vi "BBO2.vi"(6 "시작시간 값":u32, 8 "ROI 2":T1={"Global Rectangle"=[482, 445, 741, 571], "Contours"=[{"Contour Type"=0, "ROI Type"=3, "Points"=[482, 445, 741, 571]}]}, 9 "카메라 X":dbl=22.0, 10 "핀간격":dbl=40.0, 11 "클러스터":T2={{"정지할 차이값"=0.08, "흰색과 밖 차이값"=0.15, "흰/검 반 값 "=0.3}, {"4: 오른각도"=122.0, "4: 뒷쪽각도"=0.0, "5: 오른각도"=120.0, "5: 앞쪽각도"=245.0, "6: 왼쪽각도"=245.0, "6: 앞쪽각도"=120.0}, {"2: 공각도"=233.0, "2: 굴릴각도"=60.0}}) -> (3 "ROI":T1={"Global Rectangle"=[536, 448, 795, 574], "Contours"=[{"Contour Type"=0, "ROI Type"=3, "Points"=[536, 448, 795, 574]}]})   [LabVIEW 2014]
doc: "The myRIO Project template acquires acceleration data from the onboard accelerometer and displays the changes of acceleration values in a waveform chart."
uses:
  <vilib>/userdefined/High Color/IMAQdx.ctl
  <vilib>/vision/driver/NI_Vision_Acquisition_Software.lvlib
  <vilib>/vision/NI_Vision_Development_Module.lvlib
panel:
  out "시간체크":u32=10797
  in  "Range":cluster{"Lower value":sgl, "Upper value":sgl}={"Lower value"=128.0, "Upper value"=255.0} {"Upper value" format="%.2f"; "Lower value" format="%.2f"}
  in  "조정":dbl=100.0
  in  "수평(뒤로) 초":u32=150
  out "Number of Particles":i32=4
  in  "Local":T3={"Object Type"=0, "Method"=1, "Niblack Deviation Factor"=1.0, "Window"={"Width"=20, "Height"=20}} {"Niblack Deviation Factor" min=0.0 max=1.0 format="%.2f"; "Method" items=["Niblack", "Background Correction"]; "Object Type" items=["Bright Objects", "Dark Objects"]}
  out "숫자형 컨트롤":i32=11
  out "볼링핀을찾았는가":bool=TRUE
  in  "공 굴릴 범위":dbl=5.0
  in  "작게 움직이는 범위":dbl=500.0
  in  "좌우모터":i16=25
  out "Image 2":T4(plugin-control)
  out "Image":T4(plugin-control)
  # "Control Motor"
  # "Read Encoder"
  # "중간 22"
  # "25"
  # "1,3핀 12"
  # "1일때 + 0일때 -"
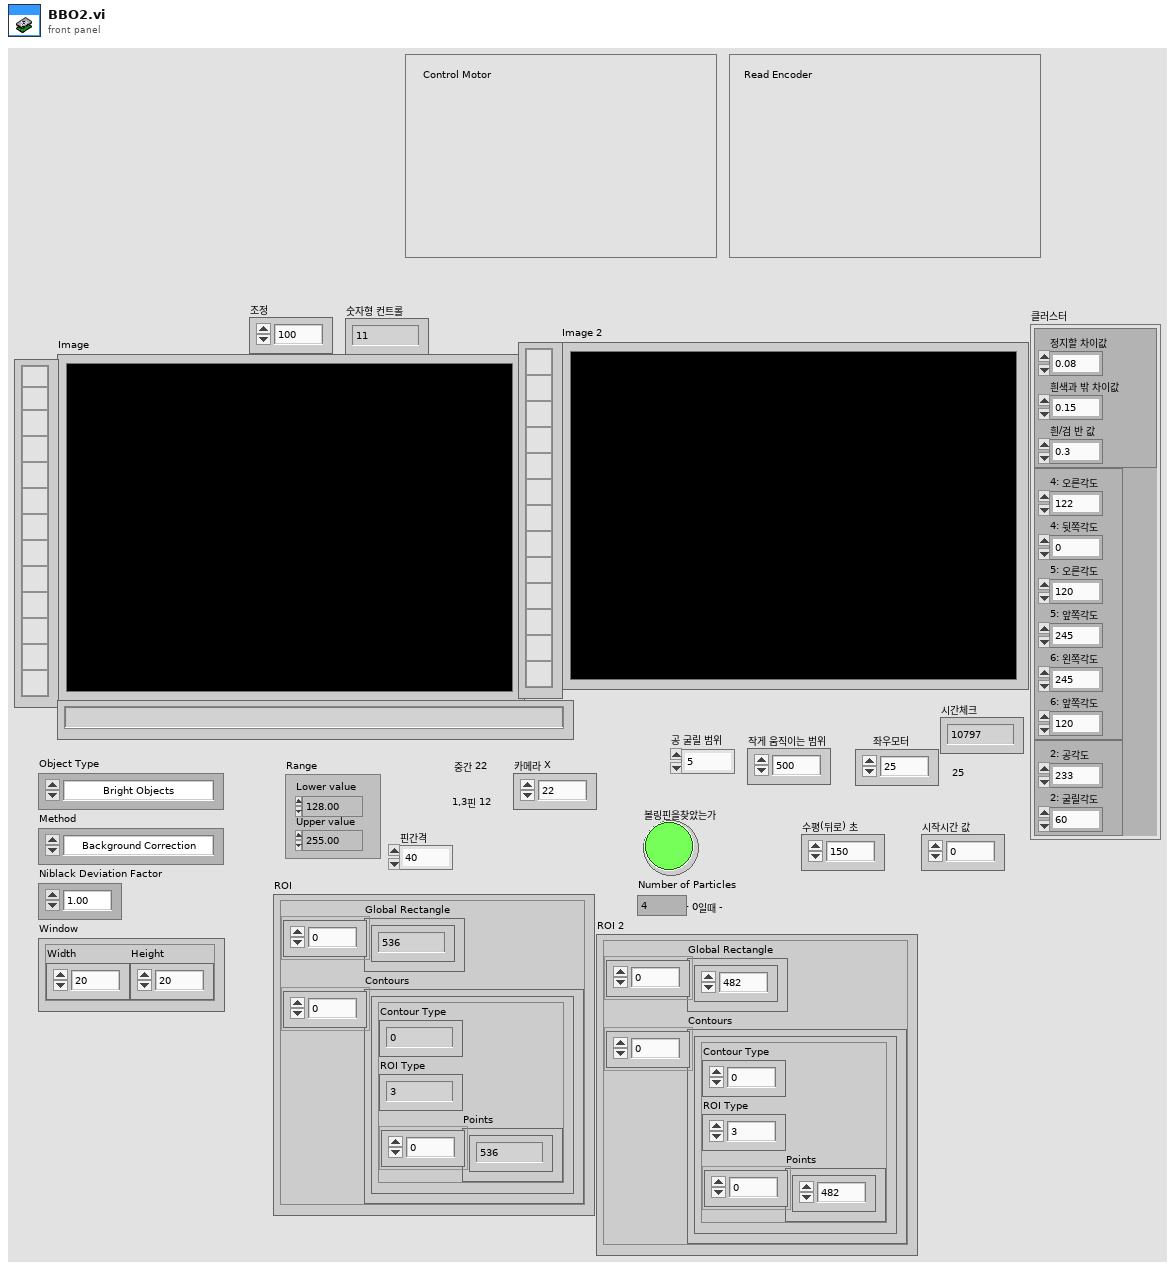
[diagram p1: front panel]
types:
  T1 = cluster{"Global Rectangle":i32[], "Contours":cluster{"Contour Type":u32, "ROI Type":u32, "Points":i32[]}[]}
  T2 = cluster{cluster{"정지할 차이값":dbl, "흰색과 밖 차이값":dbl, "흰/검 반 값 ":dbl}, cluster{"4: 오른각도":dbl, "4: 뒷쪽각도":dbl, "5: 오른각도":dbl, "5: 앞쪽각도":dbl, "6: 왼쪽각도":dbl, "6: 앞쪽각도":dbl}, cluster{"2: 공각도":dbl, "2: 굴릴각도":dbl}}
  T3 = cluster{"Object Type":u32, "Method":u32, "Niblack Deviation Factor":dbl, "Window":cluster{"Width":i32, "Height":i32}}
  T4 = typedef "IMAQ Image.ctl" = refnum<image>
  T5 = typedef "IMAQdx.ctl" = refnum<k21>
  T6 = typedef "IMAQ Rectangle" = cluster{"Left":i32, "Top":i32, "Right":i32, "Bottom":i32, "Rotation":dbl}
  T7 = cluster{"Niblack Deviation Factor":dbl, "Niblack Deviation Factor":dbl}
  T8 = typedef "Image Type" = u32
  T9 = cluster{"Area":dbl, "Number of Holes":dbl, "Bounding Rect":cluster{"Left":dbl, "Top":dbl, "Right":dbl, "Bottom":dbl}, "Center of Mass":cluster{"X":dbl, "Y":dbl}, "Orientation":dbl, "Dimensions":cluster{"Width":dbl, "Height":dbl}}[]
  T10 = cluster{"Left":dbl, "Top":dbl, "Right":dbl, "Bottom":dbl}
  T11 = typedef "ROI Descriptor" = cluster{"Global Rectangle":i32[], "Contours":cluster{"ID":enum32{"External", "Internal"}, "Type":u32, "Coordinates":i32[]}[]}
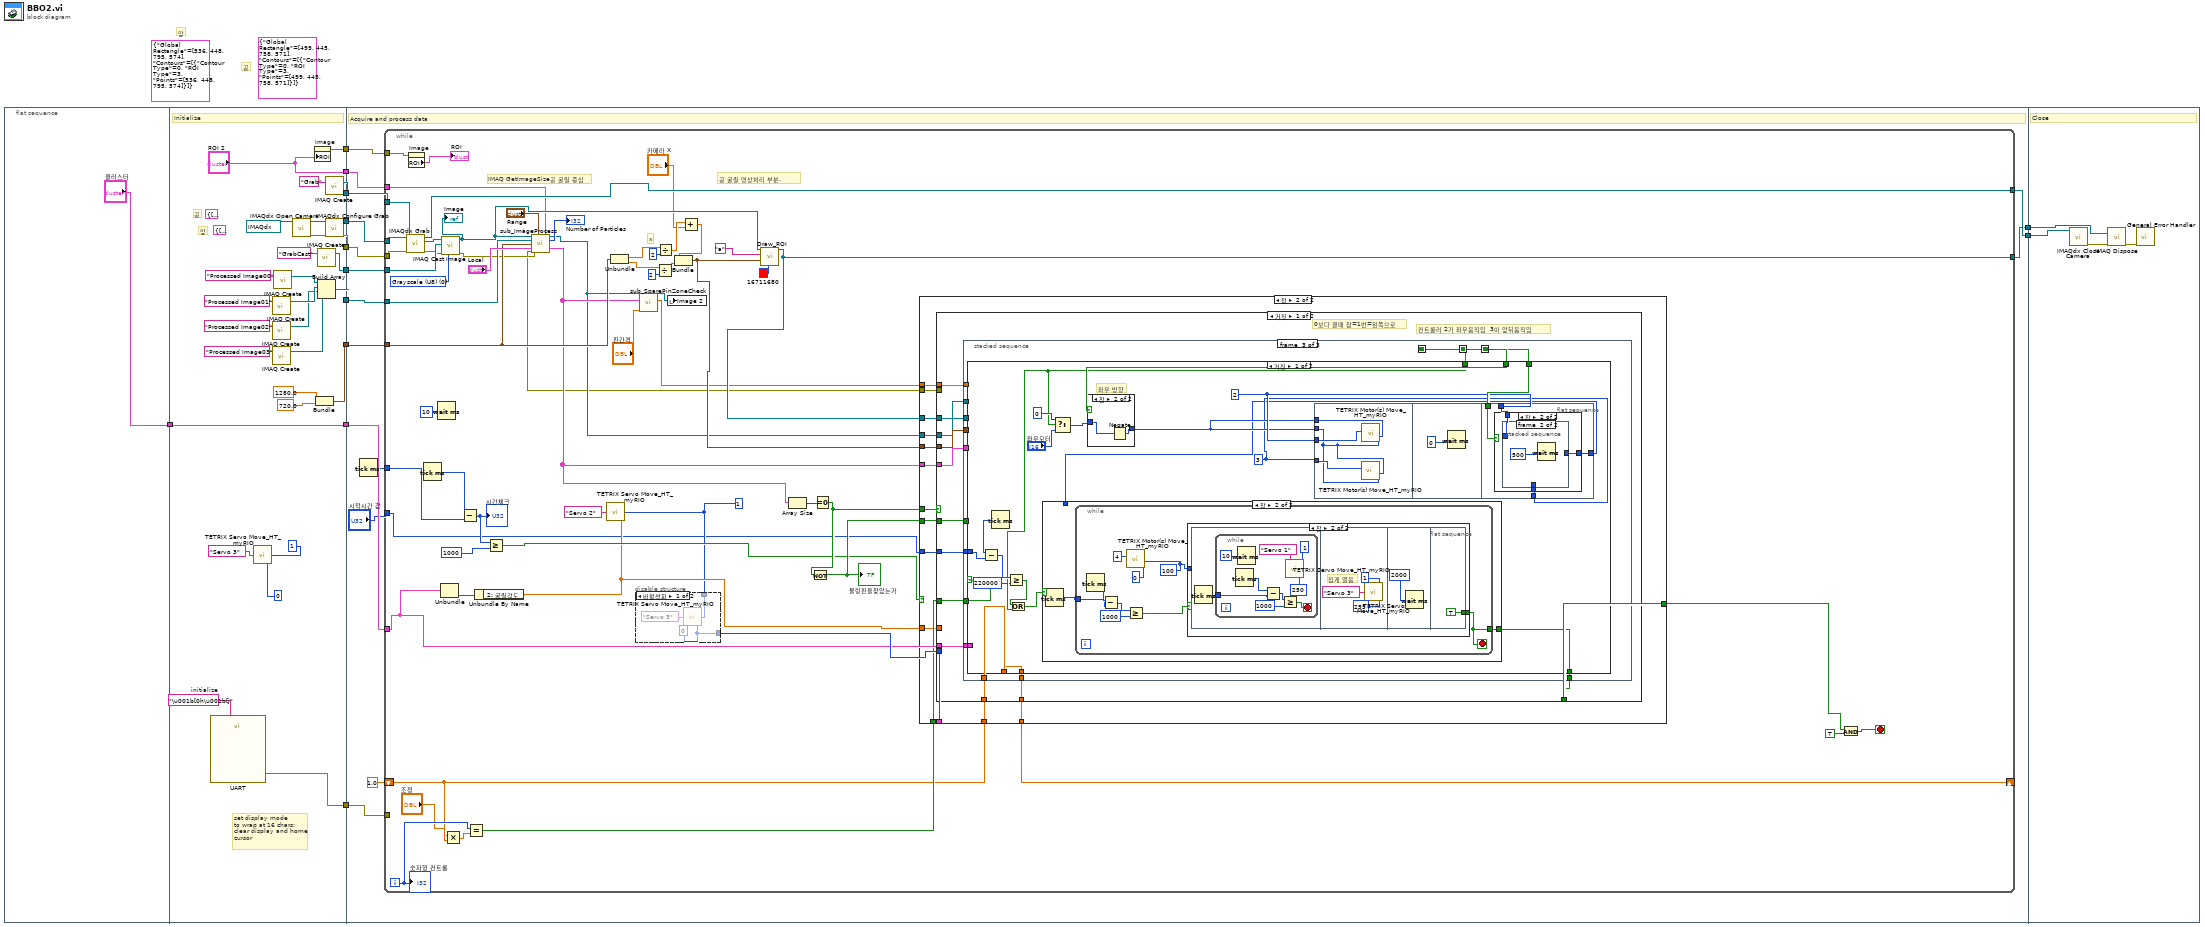
[diagram p0: block diagram]
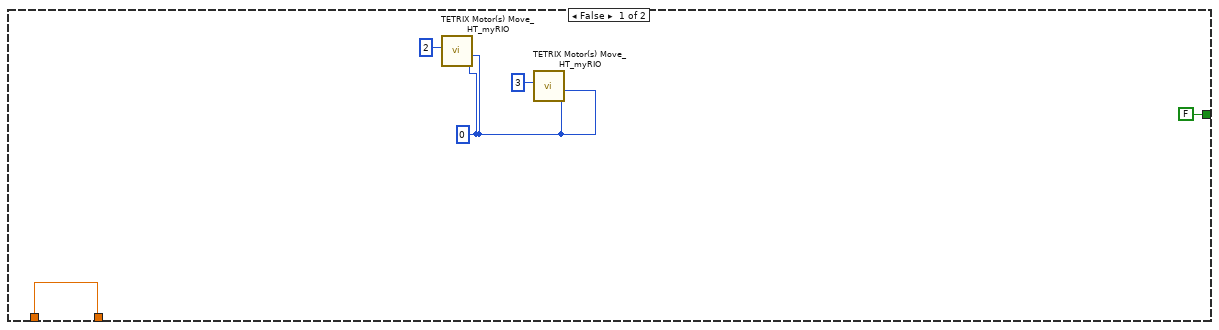
[diagram p3: hidden frame]
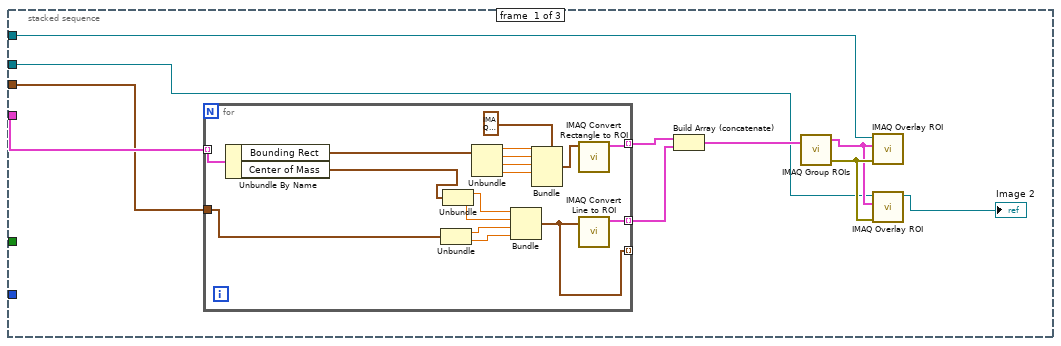
[diagram p4: hidden frame]
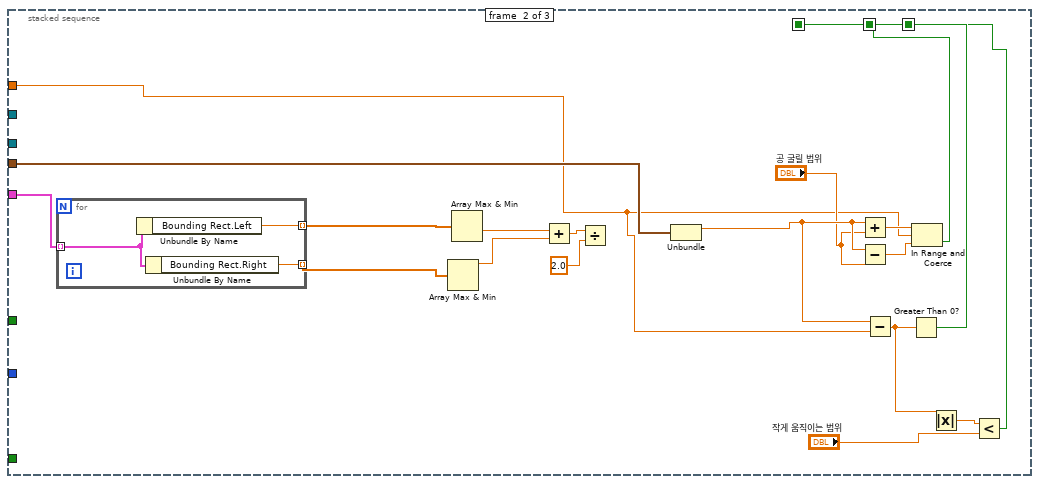
[diagram p5: hidden frame]
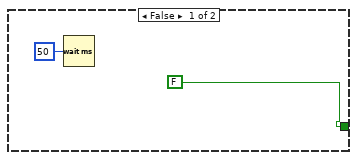
[diagram p6: hidden frame]
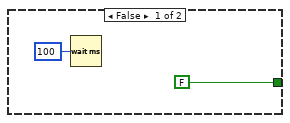
[diagram p7: hidden frame]
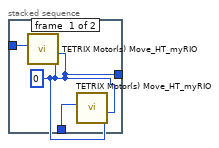
[diagram p9: hidden frame]
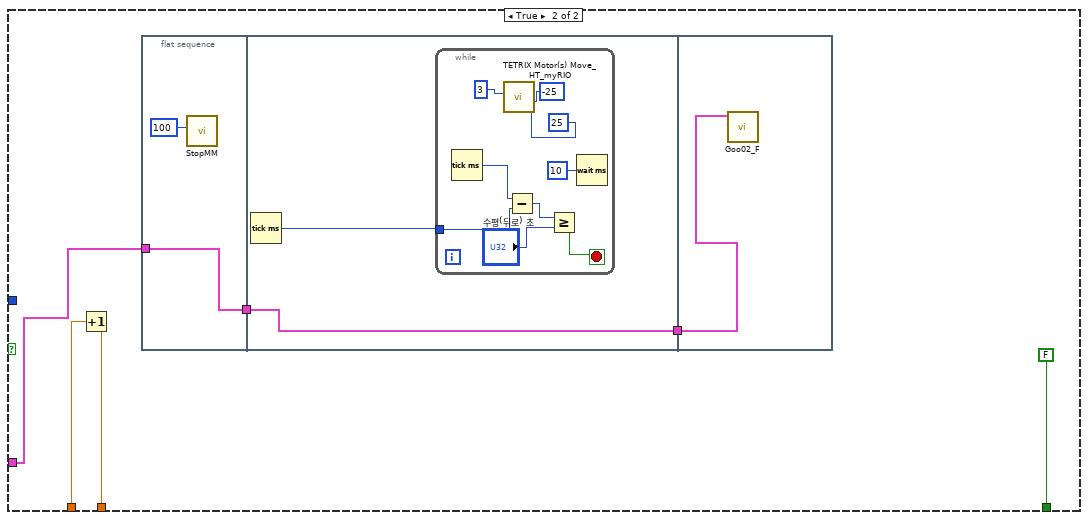
[diagram p11: hidden frame]
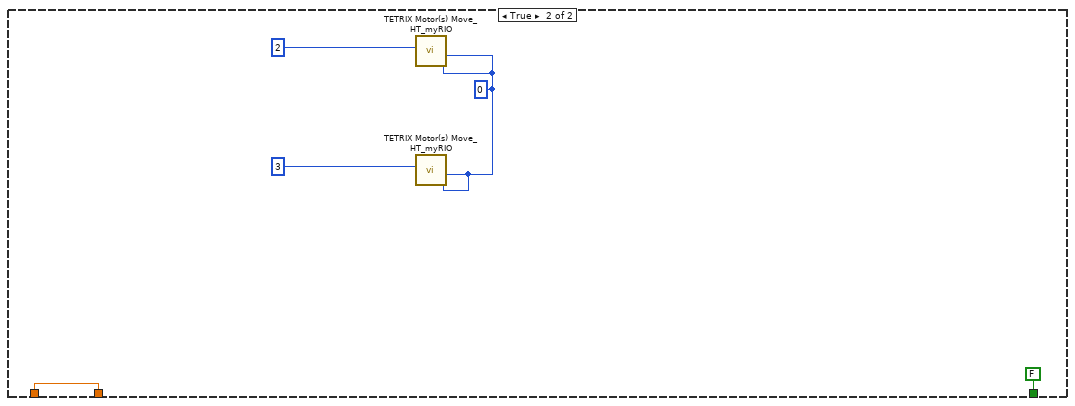
[diagram p12: hidden frame]
diagram:
  (unwired) T1 {"Global Rectangle"=[499, 445, 758, 571], "Contours"=[{"Contour Type"=0, "ROI Type"=3, "Points"=[499, 445, 758, 571]}]} ("ROI")
  (unwired) T1 {"Global Rectangle"=[536, 448, 795, 574], "Contours"=[{"Contour Type"=0, "ROI Type"=3, "Points"=[536, 448, 795, 574]}]} ("ROI")
  # "공"
  # "앞"
  n1 = flat-sequence {
    tunnel: ["클러스터"] -> w3
    tunnel: [w40] -> w13
    tunnel: [w39] -> w12
    tunnel: [w38] -> w11
    tunnel: [w26] -> w10
    tunnel: [w36] -> w9
    tunnel: [w33] -> w6
    tunnel: [w30] -> w5
    tunnel: [w21] -> w4
    tunnel: w3 -> [w21]
    tunnel: ["ROI 2"] -> w2
    tunnel: [w19] -> w1
    tunnel: w13 -> [w58]
    tunnel: w12 -> [w57]
    tunnel: w11 -> [w56]
    tunnel: [w53] -> w8
    tunnel: [w55] -> w7
    tunnel: w10 -> [w54]
    tunnel: w9 -> [w52]
    tunnel: w6 -> [w51]
    tunnel: w5 -> [w50]
    tunnel: w4 -> [w48]
    tunnel: w2 -> [w46]
    tunnel: w1 -> [w47]
    tunnel: w8 -> [w308]
    tunnel: w7 -> [w307]
    frame #0 {
    }
    frame #1 {
      (unwired) T1 {"Global Rectangle"=[536, 448, 795, 574], "Contours"=[{"Contour Type"=0, "ROI Type"=3, "Points"=[536, 448, 795, 574]}]} ("ROI")
      (unwired) T1 {"Global Rectangle"=[499, 445, 758, 571], "Contours"=[{"Contour Type"=0, "ROI Type"=3, "Points"=[499, 445, 758, 571]}]} ("ROI")
      w35 = "\u001b[0h\u001b[j"  # initialize
      # "공"
      # "앞"
      # "set display mode\nto wrap at 16 chars;\nclear display and home\ncursor"
      # "Initialize"
      n2 = call "UART"("Characters to Write"=w35) -> ("error out"=w36:errorcluster)  [unwired: 25 in, 1 out]
      n3 = call <vilib>:"TETRIX Servo Move_HT_myRIO.vi"("Servo Position (0 - 255)"=u8 0, "Controller Daisy Chain Position (1 - 4)"=u8 1, "Select Servo"="Servo 3") -> ()  [unwired: 2 in, 1 out]
      n4 = call "IMAQ Create"("Image Name"="Processed Image01") -> ("New Image"=w27:T4)  [unwired: 3 in, 2 out]
      n5 = call "IMAQ Create"("Image Name"="Processed Image02") -> ("New Image"=w23:T4)  [unwired: 3 in, 2 out]
      n6 = call "IMAQ Create"("Image Name"="Processed Image03") -> ("New Image"=w22:T4)  [unwired: 3 in, 2 out]
      n7 = call "IMAQ Create"("Image Name"="Processed Image00") -> ("New Image"=w28:T4)  [unwired: 3 in, 2 out]
      n8 = call <vilib>:"IMAQdx Open Camera.vi"("Session In"=T5 "cam1") -> ("error out"=w43:errorcluster, "Session Out"=w42:T5)  [unwired: 2 in, 7 out]
      n9 = property on="Image" class="ImageControl"("ROI"="ROI 2") -> (error out=w19:errorcluster)  [unwired: 2 in, 1 out]
      n10 = Bundle("Niblack Deviation Factor"=1280.0, "Niblack Deviation Factor"=720.0) -> (w30:T7)  [unwired: 1 in]
      n11 = call "IMAQ Create"("Image Name"="GrabCast") -> ("New Image"=w33:T4)  [unwired: 3 in, 2 out]
      n12 = Build Array(w28, w27, w23, w22) -> (w26:T4[])
      n13 = call "IMAQ Create"("Image Name"="Grab") -> ("New Image"=w40:T4)  [unwired: 3 in, 2 out]
      n14 = call <vilib>:"IMAQdx Configure Grab.vi"("error in"=w43, "Session In"=w42) -> ("error out"=w38:errorcluster, "Session Out"=w39:T5)  [unwired: 8 out]
    }
    frame #2 {
      # "Acquire and process data"
      n15 = Tick Count (ms)() -> (millisecond timer value=w44:u32)
      n16 = while {
        tunnel: [w116] -> w55
        tunnel: w56 -> [w118]
        tunnel: w57 -> [w119]
        tunnel: w58 -> [w117]
        tunnel: w54 -> [w98]
        tunnel: [w108] -> w53
        tunnel: w52 -> [_]
        tunnel: w51 -> [w103]
        tunnel: w50 -> [w97]
        shift-right: [w90] -> _
        shift-left: 1.0 -> [w88]
        tunnel: w48 -> [w67]
        tunnel: w47 -> [w75]
        tunnel: w46 -> [w74]
        tunnel: "시작시간 값" -> [w60]
        tunnel: w44 -> [w59]
        i -> [w92]
        stop <- w106 stop-if-true
        w82 = T8 0 items=["Grayscale (U8)", "Grayscale (I16)", "Grayscale (SGL)", "Complex (CSG)", "RGB (U32)", "HSL (U32)", "RGB (U64)", "Grayscale (U16)"] ("Image Type")
        w64 = u8 1 ("Controller Daisy Chain Position (1 - 4)")
        # "공 굴릴 영상처리 부분."
        # "IMAQ GetImageSize공 굴릴 중심"
        # "x"
        n17 = call <vilib>:"IMAQdx Grab.vi"("error in"=w118, "Image In"=w117, "Session In"=w119) -> ("error out"=w102:errorcluster, "Image Out"=w104:T4, "Session Out"=w116:T5)  [unwired: 1 in, 5 out]
        n18 = property on="Image" class="ImageControl"(error in=w75) -> ("ROI"=→"ROI":T1)  [unwired: 1 in, 2 out]
        n19 = Tick Count (ms)() -> (millisecond timer value=w71:u32)
        n20 = Wait (ms)(milliseconds to wait=u32 10 ("대기 시간(ms)")) -> ()  [unwired: 1 out]
        n21 = Unbundle(w67) -> (w66:cluster{"2: 공각도":dbl, "2: 굴릴각도":dbl})  [unwired: 2 out]
        n22 = call "IMAQ Cast Image"("Image Type"=w82, "error in (no error)"=w102, "Image Dst"=w103, "Image Src"=w104) -> ("error out"=w81:errorcluster, "Image Dst Out"=w100:T4)  [unwired: 6 in]
        "Image" <- w100
        n23 = Multiply(x="조정", y=w88) -> (x*y=w91:dbl)
        n24 = Subtract(x=w71, y=w59) -> (x-y=w70:u32)
        "시간체크" <- w70
        n25 = Equal?(x=w92, y=w91) -> (x = y?=w89:bool)
        n26 = Unbundle By Name(w66) -> ("2: 굴릴각도"=w65:dbl)
        n27 = Greater Or Equal?(x=w70, y=u32 1000) -> (x >= y?=w68:bool)
        n28 = call "sub_ImageProcess.vi"("참조 번호 입력"=w100, "Range"="Range", "ROI"=w74, "배열"=w98, "클러스터"=w97, "Local"="Local", "에러 입력(에러 없음)"=w81) -> ("참조 번호 출력"=w77:T4, "Number of Particles"=→"Number of Particles":i32, "Particle Reports (Pixels)"=w86:T9, "error out"=w72:errorcluster)  [unwired: 5 in]
        n29 = call <vilib>:"TETRIX Servo Move_HT_myRIO.vi"("Servo Position (0 - 255)"=w65, "Controller Daisy Chain Position (1 - 4)"=w64, "Select Servo"="Servo 2") -> ()  [unwired: 2 in, 1 out]
        n30 = Unbundle(w97) -> ("Niblack Deviation Factor"=w96:dbl, "Niblack Deviation Factor"=w95:dbl)
        n31 = disable-structure shown="비활성화" {
          disable-tunnel: [w121 _] -> w83
          disable-tunnel: w64 -> [w120 _]
          frame Disabled {
            w121 = u8 0 ("Servo Position (0 - 255)")
            n32 = call <vilib>:"TETRIX Servo Move_HT_myRIO.vi"("Servo Position (0 - 255)"=w121, "Controller Daisy Chain Position (1 - 4)"=w120, "Select Servo"="Servo 3") -> ()  [unwired: 2 in, 1 out]
          }
          frame Enabled {
          }
        }
        n33 = call "sub_SparePinZoneCheck.vi"("핀간격"="핀간격", "Particle Reports (Pixels)"=w86, "참조 번호 입력"=w77) -> ("숫자형"=w84:dbl, "참조 번호 출력"=w85:T4)  [unwired: 7 in]
        n34 = Divide(x=w95, y=2) -> (x/y=w113:dbl)
        n35 = Divide(x=w96, y=2) -> (x/y=w94:dbl)
        n36 = local write "Image 2"(w85) -> ()
        n37 = Add(x=w94, y="카메라 X") -> (x+y=w93:dbl)
        n38 = Bundle(w93, w113) -> (w110:cluster{dbl, dbl})  [unwired: 1 in]
        n39 = call "Draw_ROI.vi"("Color"=u32 16711680, "클러스터"=w110, "Group"="a", "참조 번호 입력"=w100) -> ("참조 번호 출력"=w108:T4)  [unwired: 7 in]
        n40 = Array Size(array=w86) -> (size(s)=w78:i32)
        n41 = Equal To 0?(x=w78) -> (x = 0?=w80:bool)
        n42 = Not(x=w80) -> (.not. x?=w79:bool)
        "볼링핀을찾았는가" <- w79
        n43 = case shown="참" w68 {
          tunnel: w110 -> [_ w143]
          tunnel: w108 -> [_ w142]
          tunnel: [FALSE w141] -> w107
          tunnel: [w124 w140] -> w90
          tunnel: w89 -> [_ w139]
          tunnel: w88 -> [w124 w138]
          tunnel: w86 -> [_ w137]
          tunnel: w84 -> [_ w136]
          tunnel: w83 -> [_ w135]
          tunnel: w67 -> [_ w134]
          tunnel: w80 -> [_ w133]
          tunnel: w79 -> [_ w132]
          tunnel: w77 -> [_ w131]
          tunnel: w72 -> [_ w130]
          tunnel: w65 -> [_ w129]
          tunnel: w60 -> [_ w128]
          frame False {
            w125 = i8 0 ("Motor 1 Power (-100 to 100)\n0 = Stop/Brake\n-128 = Stop/Coast")
            n44 = call <vilib>:"TETRIX Motor(s) Move_HT_myRIO.vi"("Motor 2 Power (-100 to 100)\n0 = Stop/Brake\n-128 = Stop/Coast"=w125, "Motor 1 Power (-100 to 100)\n0 = Stop/Brake\n-128 = Stop/Coast"=w125, "Controller Daisy Chain Position: 1 - 4"=u8 2) -> ()  [unwired: 6 in, 1 out]
            n45 = call <vilib>:"TETRIX Motor(s) Move_HT_myRIO.vi"("Motor 2 Power (-100 to 100)\n0 = Stop/Brake\n-128 = Stop/Coast"=w125, "Motor 1 Power (-100 to 100)\n0 = Stop/Brake\n-128 = Stop/Coast"=w125, "Controller Daisy Chain Position: 1 - 4"=u8 3) -> ()  [unwired: 6 in, 1 out]
          }
          frame True {
            n46 = case shown="거짓" w133 {
              tunnel: w137 -> [w155 _]
              tunnel: w143 -> [w154 _]
              tunnel: w131 -> [w153 _]
              tunnel: w142 -> [w152 _]
              tunnel: [w151 FALSE] -> w141
              tunnel: w130 -> [_ _]
              tunnel: [w150 w302] -> w140
              tunnel: w139 -> [w149 _]
              tunnel: w138 -> [w148 w302]
              tunnel: w136 -> [w147 _]
              tunnel: w135 -> [_ _]
              tunnel: w134 -> [w146 _]
              tunnel: w132 -> [w145 _]
              tunnel: w129 -> [_ _]
              tunnel: w128 -> [w144 _]
              frame False {
                # "0보다 클때 참=1번=왼쪽으로"
                # "컨트롤러 2가 좌우움직임  3이 앞뒤움직임"
                n47 = stacked-sequence {
                  seq-local: [_ w185 _] -> [_ _ w211]
                  seq-local: [_ w192 _] -> [_ _ w213]
                  seq-local: [_ w188 _] -> [_ _ w212]
                  tunnel: w155 -> [w160 w195 _]
                  tunnel: w154 -> [w157 w194 _]
                  tunnel: w153 -> [w159 _ _]
                  tunnel: w152 -> [w158 _ _]
                  tunnel: [_ _ w210] -> w151
                  tunnel: [_ _ w209] -> w150
                  tunnel: w149 -> [_ _ w208]
                  tunnel: w148 -> [_ _ w207]
                  tunnel: w147 -> [_ w186 _]
                  tunnel: w146 -> [_ _ w206]
                  tunnel: w145 -> [_ _ _]
                  tunnel: w144 -> [_ _ w205]
                  frame #0 {
                    n48 = for {
                      tunnel: w160 -> [w182] mode=indexing
                      tunnel: [w174] -> w162 mode=indexing
                      tunnel: w157 -> [w170]
                      tunnel: [w167] -> w164 mode=indexing
                      tunnel: [w166] -> _ mode=indexing
                      n49 = Unbundle By Name(w182) -> ("Bounding Rect"=w180:T10, "Center of Mass"=w173:cluster{"X":dbl, "Y":dbl})
                      n50 = Unbundle(w170) -> (w169:dbl, w168:dbl)
                      n51 = Unbundle(w173) -> ("X"=w172:dbl, "Y"=w171:dbl)
                      n52 = Unbundle(w180) -> ("Left"=w179:dbl, "Top"=w178:dbl, "Right"=w177:dbl, "Bottom"=w176:dbl)
                      n53 = Bundle("X"=w172, "Y"=w171, w169, w168) -> (w166:cluster{"X":dbl, "Y":dbl, dbl, dbl})  [unwired: 1 in]
                      n54 = Bundle(cluster=T6 {"Left"=0, "Top"=0, "Right"=0, "Bottom"=0, "Rotation"=0.0} ("Rectangle"), "Left"=w179, "Top"=w178, "Right"=w177, "Bottom"=w176) -> (w175:T6)  [unwired: 1 in]
                      n55 = call "IMAQ Convert Rectangle to ROI"("Rectangle"=w175) -> ("ROI Descriptor"=w174:T11)  [unwired: 8 in, 1 out]
                      n56 = call "IMAQ Convert Line to ROI"("Line"=w166) -> ("ROI Descriptor"=w167:T11)  [unwired: 8 in, 1 out]
                    }
                    n57 = Build Array (concatenate)(w162, w164) -> (w163:T11[])
                    n58 = call "IMAQ Group ROIs"("ROI Descriptors"=w163) -> ("error out"=w165:errorcluster, "ROI Descriptor out"=w161:T11)  [unwired: 1 in, 2 out]
                    n59 = call "IMAQ Overlay ROI"("error in (no error)"=w165, "ROI Descriptor"=w161, "Image"=w158) -> ()  [unwired: 3 in, 6 out]
                    n60 = call "IMAQ Overlay ROI"("error in (no error)"=w165, "ROI Descriptor"=w161, "Image"=w159) -> ("Image Out"=→"Image 2":T4)  [unwired: 3 in, 5 out]
                  }
                  frame #1 {
                    n61 = for {
                      tunnel: w195 -> [w204] mode=indexing
                      tunnel: [w203] -> w200 mode=indexing
                      tunnel: [w202] -> w201 mode=indexing
                      n62 = Unbundle By Name(w204) -> ("Bounding Rect.Left"=w203:dbl)
                      n63 = Unbundle By Name(w204) -> ("Bounding Rect.Right"=w202:dbl)
                    }
                    n64 = Array Max & Min(array=w201) -> (max value=w183:dbl)  [unwired: 3 out]
                    n65 = Array Max & Min(array=w200) -> (min value=w184:dbl)  [unwired: 3 out]
                    n66 = Add(x=w184, y=w183) -> (x+y=w196:dbl)
                    n67 = Divide(x=w196, y=2.0) -> ()  [unwired: 1 out]
                    n68 = Unbundle(w194) -> (w193:dbl)  [unwired: 1 out]
                    n69 = Add(x=w193, y="공 굴릴 범위") -> (x+y=w198:dbl)
                    n70 = Subtract(x=w193, y="공 굴릴 범위") -> (x-y=w199:dbl)
                    n71 = Subtract(x=w193, y=w186) -> (x-y=w191:dbl)
                    n72 = Greater Than 0?(x=w191) -> (x > 0?=w192:bool)
                    n73 = In Range and Coerce(upper limit=w198, x=w186, lower limit=w199) -> (In Range?=w185:bool)  [unwired: 1 out]
                    n74 = Absolute Value(x=w191) -> (abs(x)=w190:dbl)
                    n75 = Less?(x=w190, y="작게 움직이는 범위") -> (x < y?=w188:bool)
                  }
                  frame #2 {
                    n76 = case shown="거짓" w208 {
                      tunnel: w213 -> [w231 _]
                      tunnel: w212 -> [w230 _]
                      tunnel: w211 -> [w216 _]
                      tunnel: [w221 FALSE] -> w210
                      tunnel: [w225 w286] -> w209
                      tunnel: w207 -> [w225 w285]
                      tunnel: w206 -> [_ w282]
                      tunnel: w205 -> [w218 _]
                      frame False {
                        w223 = u8 3 ("Controller 2")
                        w227 = u8 2 ("Controller 2")
                        # "좌우 방향"
                        n77 = Tick Count (ms)() -> (millisecond timer value=w219:u32)
                        n78 = Subtract(x=w219, y=w218) -> (x-y=w220:u32)
                        n79 = Greater Or Equal?(x=w220, y=u32 220000) -> (x >= y?=w217:bool)
                        n80 = Or(x=w217, y=w216) -> (x .or. y?=w215:bool)
                        n81 = case shown="참" w215 {
                          tunnel: w222 -> [_ _]
                          tunnel: [FALSE w234] -> w221
                          frame False {
                            n82 = Wait (ms)(milliseconds to wait=u32 50 ("대기 시간(ms)")) -> ()  [unwired: 1 out]
                          }
                          frame True {
                            n83 = Tick Count (ms)() -> (millisecond timer value=w235:u32)
                            n84 = while {
                              tunnel: w235 -> [w241]
                              tunnel: [w237] -> w234
                              stop <- w237 stop-if-true
                              w236 = i8 100 ("Motor 1 Power (-100 to 100)\n0 = Stop/Brake\n-128 = Stop/Coast")
                              n85 = Tick Count (ms)() -> (millisecond timer value=w242:u32)
                              n86 = Subtract(x=w242, y=w241) -> (x-y=w240:u32)
                              n87 = call <vilib>:"TETRIX Motor(s) Move_HT_myRIO.vi"("Motor 2 Power (-100 to 100)\n0 = Stop/Brake\n-128 = Stop/Coast"=i8 0 ("Motor 2 Power (-100 to 100)\n0 = Stop/Brake\n-128 = Stop/Coast"), "Motor 1 Power (-100 to 100)\n0 = Stop/Brake\n-128 = Stop/Coast"=w236, "Controller Daisy Chain Position: 1 - 4"=u8 4) -> ()  [unwired: 6 in, 1 out]
                              n88 = Greater Or Equal?(x=w240, y=u32 1000) -> (x >= y?=w239:bool)
                              n89 = case shown="참" w239 {
                                tunnel: w236 -> [_ _]
                                tunnel: [FALSE w247] -> w237
                                frame False {
                                n90 = Wait (ms)(milliseconds to wait=u32 100 ("대기 시간(ms)")) -> ()  [unwired: 1 out]
                                }
                                frame True {
                                n91 = flat-sequence {
                                tunnel: [TRUE] -> w247
                                frame #0 {
                                n92 = Tick Count (ms)() -> (millisecond timer value=w248:u32)
                                n93 = while {
                                tunnel: w248 -> [w256]
                                stop <- w254 stop-if-true
                                n94 = Tick Count (ms)() -> (millisecond timer value=w257:u32)
                                n95 = Wait (ms)(milliseconds to wait=u32 10 ("대기 시간(ms)")) -> ()  [unwired: 1 out]
                                n96 = Subtract(x=w257, y=w256) -> (x-y=w255:u32)
                                n97 = Greater Or Equal?(x=w255, y=u32 1000) -> (x >= y?=w254:bool)
                                n98 = call <vilib>:"TETRIX Servo Move_HT_myRIO.vi"("Servo Position (0 - 255)"=u8 250, "Controller Daisy Chain Position (1 - 4)"=u8 1, "Select Servo"="Servo 1") -> ()  [unwired: 2 in, 1 out]
                                }
                                }
                                frame #1 {
                                # "집게 열음"
                                n99 = call <vilib>:"TETRIX Servo Move_HT_myRIO.vi"("Servo Position (0 - 255)"=u8 255, "Controller Daisy Chain Position (1 - 4)"=u8 1, "Select Servo"="Servo 3") -> ()  [unwired: 2 in, 1 out]
                                }
                                frame #2 {
                                n100 = Wait (ms)(milliseconds to wait=u32 2000 ("대기 시간(ms)")) -> ()  [unwired: 1 out]
                                }
                                frame #3 {
                                }
                                }
                                }
                              }
                            }
                          }
                        }
                        n101 = Select(t=i8 0 ("Motor 2 Power (-100 to 100)\n0 = Stop/Brake\n-128 = Stop/Coast"), s=w216, f="좌우모터") -> (s? t:f=w229:i16)
                        n102 = case shown="참" w231 {
                          tunnel: w229 -> [w279 w281]
                          tunnel: [w279 w280] -> w224
                          frame False {
                          }
                          frame True {
                            n103 = Negate(x=w281) -> (-x=w280:i16)
                          }
                        }
                        n104 = flat-sequence {
                          tunnel: w227 -> [w266]
                          tunnel: w224 -> [w265]
                          tunnel: w224 -> [w263]
                          tunnel: w223 -> [w264]
                          tunnel: w227 -> [w271]
                          tunnel: w230 -> [w270]
                          tunnel: [w269] -> w222
                          tunnel: w223 -> [w268]
                          frame #0 {
                            n105 = call <vilib>:"TETRIX Motor(s) Move_HT_myRIO.vi"("Motor 2 Power (-100 to 100)\n0 = Stop/Brake\n-128 = Stop/Coast"=w263, "Motor 1 Power (-100 to 100)\n0 = Stop/Brake\n-128 = Stop/Coast"=w263, "Controller Daisy Chain Position: 1 - 4"=w264) -> ()  [unwired: 6 in, 1 out]
                            n106 = call <vilib>:"TETRIX Motor(s) Move_HT_myRIO.vi"("Motor 2 Power (-100 to 100)\n0 = Stop/Brake\n-128 = Stop/Coast"=w263, "Motor 1 Power (-100 to 100)\n0 = Stop/Brake\n-128 = Stop/Coast"=w265, "Controller Daisy Chain Position: 1 - 4"=w266) -> ()  [unwired: 6 in, 1 out]
                          }
                          frame #1 {
                            n107 = Wait (ms)(milliseconds to wait=u32 0 ("대기 시간(ms)")) -> ()  [unwired: 1 out]
                          }
                          frame #2 {
                            n108 = case shown="참" w270 {
                              tunnel: w271 -> [_ w274]
                              tunnel: [_ w272] -> w269
                              tunnel: w268 -> [_ w273]
                              frame False {
                              }
                              frame True {
                                n109 = stacked-sequence {
                                tunnel: w274 -> [w277 _]
                                tunnel: w273 -> [w276 _]
                                tunnel: [w275 _] -> w272
                                frame #0 {
                                w275 = i8 0 ("Motor 2 Power (-100 to 100)\n0 = Stop/Brake\n-128 = Stop/Coast")
                                n110 = call <vilib>:"TETRIX Motor(s) Move_HT_myRIO.vi"("Motor 2 Power (-100 to 100)\n0 = Stop/Brake\n-128 = Stop/Coast"=w275, "Motor 1 Power (-100 to 100)\n0 = Stop/Brake\n-128 = Stop/Coast"=w275, "Controller Daisy Chain Position: 1 - 4"=w277) -> ()  [unwired: 6 in, 1 out]
                                n111 = call <vilib>:"TETRIX Motor(s) Move_HT_myRIO.vi"("Motor 2 Power (-100 to 100)\n0 = Stop/Brake\n-128 = Stop/Coast"=w275, "Motor 1 Power (-100 to 100)\n0 = Stop/Brake\n-128 = Stop/Coast"=w275, "Controller Daisy Chain Position: 1 - 4"=w276) -> ()  [unwired: 6 in, 1 out]
                                }
                                frame #1 {
                                n112 = Wait (ms)(milliseconds to wait=u32 500 ("대기 시간(ms)")) -> ()  [unwired: 1 out]
                                }
                                }
                              }
                            }
                          }
                        }
                      }
                      frame True {
                        n113 = Increment(x=w285) -> (x+1=w286:dbl)
                        n114 = flat-sequence {
                          tunnel: [w288] -> w283
                          tunnel: w282 -> [w288]
                          tunnel: [w290] -> w284
                          tunnel: w283 -> [w290]
                          tunnel: w284 -> [w301]
                          frame #0 {
                            n115 = call "StopMM.vi"("대기 시간(ms)"=u32 100) -> ()  [unwired: 11 in]
                          }
                          frame #1 {
                            n116 = Tick Count (ms)() -> (millisecond timer value=w291:u32)
                            n117 = while {
                              tunnel: w291 -> [w295]
                              stop <- w293 stop-if-true
                              n118 = Tick Count (ms)() -> (millisecond timer value=w296:u32)
                              n119 = call <vilib>:"TETRIX Motor(s) Move_HT_myRIO.vi"("Motor 2 Power (-100 to 100)\n0 = Stop/Brake\n-128 = Stop/Coast"=i8 25 ("Motor 2 Power (-100 to 100)\n0 = Stop/Brake\n-128 = Stop/Coast"), "Motor 1 Power (-100 to 100)\n0 = Stop/Brake\n-128 = Stop/Coast"=i8 -25 ("Motor 1 Power (-100 to 100)\n0 = Stop/Brake\n-128 = Stop/Coast"), "Controller Daisy Chain Position: 1 - 4"=u8 3) -> ()  [unwired: 6 in, 1 out]
                              n120 = Subtract(x=w296, y=w295) -> (x-y=w294:u32)
                              n121 = Greater Or Equal?(x=w294, y="수평(뒤로) 초") -> (x >= y?=w293:bool)
                              n122 = Wait (ms)(milliseconds to wait=u32 10 ("대기 시간(ms)")) -> ()  [unwired: 1 out]
                            }
                          }
                          frame #2 {
                            n123 = call "Goo02_F.vi"("클러스터"=w301) -> ()  [unwired: 11 in]
                          }
                        }
                      }
                    }
                  }
                }
              }
              frame True {
                w304 = 0
                n124 = call <vilib>:"TETRIX Motor(s) Move_HT_myRIO.vi"("Motor 2 Power (-100 to 100)\n0 = Stop/Brake\n-128 = Stop/Coast"=w304, "Motor 1 Power (-100 to 100)\n0 = Stop/Brake\n-128 = Stop/Coast"=w304, "Controller Daisy Chain Position: 1 - 4"=u8 2) -> ()  [unwired: 6 in, 1 out]
                n125 = call <vilib>:"TETRIX Motor(s) Move_HT_myRIO.vi"("Motor 2 Power (-100 to 100)\n0 = Stop/Brake\n-128 = Stop/Coast"=w304, "Motor 1 Power (-100 to 100)\n0 = Stop/Brake\n-128 = Stop/Coast"=w304, "Controller Daisy Chain Position: 1 - 4"=u8 3) -> ()  [unwired: 6 in, 1 out]
              }
            }
          }
        }
        n126 = And(x=w107, y=TRUE) -> (x .and. y?=w106:bool)
        "숫자형 컨트롤" <- w92
      }
    }
    frame #3 {
      # "Close"
      n127 = call <vilib>:"IMAQdx Close Camera.vi"("Session In"=w307) -> ("error out"=w310:errorcluster)  [unwired: 1 in, 9 out]
      n128 = call "IMAQ Dispose"("Image"=w308, "error in (no error)"=w310) -> ("error out"=w309:errorcluster)  [unwired: 4 in]
      n129 = call <vilib>:"General Error Handler.vi"("error in (no error)"=w309) -> ()  [unwired: 2 in, 13 out]
    }
  }
